vi "Get.vi"(8 "error in (no error)":errorcluster, 11 "MicronMessage in":refnum<class "GRPCMessage.lvclass">) -> (0 "error out":errorcluster, 1 "Payload":string, 2 "Command":string, 3 "MicronMessage out":refnum<class "GRPCMessage.lvclass">)   [LabVIEW 2019, in "MicronGRPCServer.lvlib" / "GRPCMessage.lvclass"]
uses:
  GRPCMessage.lvclass
  GRPCMessage.lvclass/GRPCMessage.ctl
  Service/Generated/MicronGRPCGeneratedServer/RPC Service/MicronGRPC/MicronGRPC.lvclass
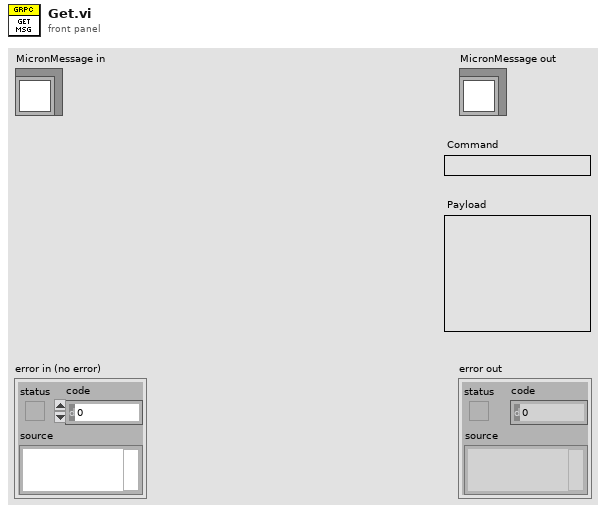
[diagram p1: front panel]
types:
  T1 = typedef "grpc-lvsupport-release.lvlib/grpcId.ctl" = u64
  T2 = typedef "MicronGRPCGeneratedServer.lvlib/micronGrpc_MessageRequest.ctl" = cluster{"command":string, "payload":string}
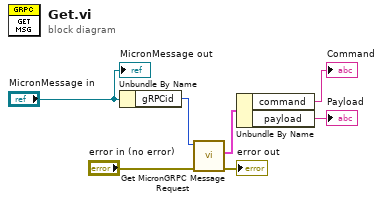
[diagram p0: block diagram]
diagram:
  n1 = Unbundle By Name("MicronMessage in") -> ("gRPCid"=w7:T1)
  n2 = call "Get MicronGRPC Message Request.vi"("error in (no error)"="error in (no error)", "gRPCid"=w7) -> ("error out"=→"error out":errorcluster, "Message Data"=w3:T2)  [unwired: 7 in, 1 out]
  n3 = Unbundle By Name(w3) -> ("command"=→"Command":string, "payload"=→"Payload":string)
  "MicronMessage out" <- "MicronMessage in"
